vi "D2Character - Accessors - Set Life Base.vi"(8 "error in (no error)":errorcluster, 10 "Life (base)":i32, 11 "D2Character in":refnum<class "D2Character.lvclass">) -> (0 "error out":errorcluster, 3 "D2Character out":refnum<class "D2Character.lvclass">)   [LabVIEW 2015, in "D2Character.lvclass"]
uses:
  D2Character.lvclass
  D2Character.lvclass/D2Character.ctl
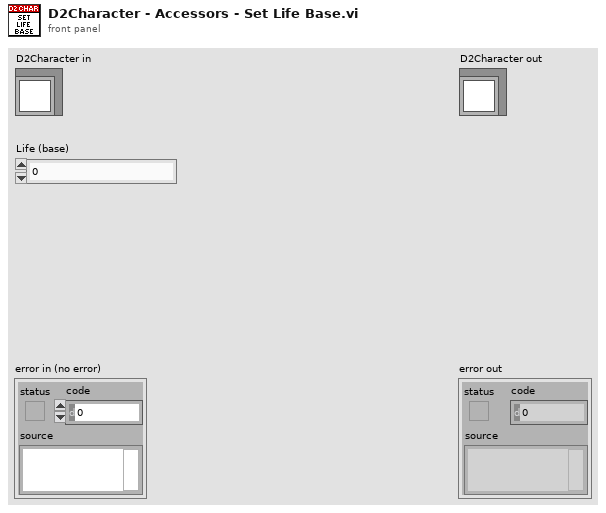
[diagram p1: front panel]
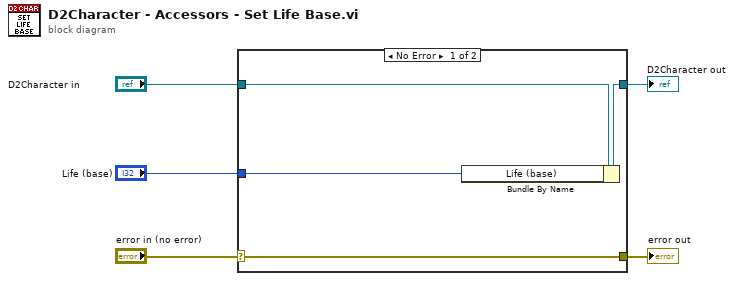
[diagram p0: block diagram]
diagram:
  n1 = case shown="No Error" "error in (no error)" {
    selector: "error in (no error)" -> [w9 w10]
    tunnel: [w9 w10] -> w4
    tunnel: [w7 w11] -> w2
    tunnel: "D2Character in" -> [w8 w11]
    tunnel: "Life (base)" -> [w6 _]
    frame No Error {
      n2 = Bundle By Name(cluster=w8, "Life (base)"=w6) -> (w7:refnum<class "D2Character.lvclass">)
    }
    frame Error {
    }
  }
  "error out" <- w4
  "D2Character out" <- w2
